vi "DP_WebView_Test.vi"() -> ()   [LabVIEW 2020, in "DP_WebView.lvclass"]
uses:
  DP_WebView.lvclass
  C:/Projects/DependencyViewer/DependencyViewer/DP_WebView_class/data/Microsoft.Web.WebView2.WinForms.dll
  data/Microsoft.Web.WebView2.WinForms.dll
panel:
  in  "Webview container":refnum<k24>(container)
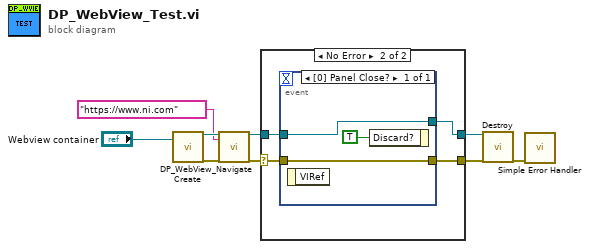
[diagram p0: block diagram]
diagram:
  n1 = call "DP_WebView_Create.vi"("Webview container"="Webview container") -> ("reference out"=w9:refnum<class "DP_WebView.lvclass">, "Error Out"=w8:errorcluster)  [unwired: 11 in, 6 out]
  n2 = call-dynamic "Navigate.vi"("reference in"=w9, "URL"="https://www.ni.com", "Error In"=w8) -> ("reference out"=w7:refnum<class "DP_WebView.lvclass">, "Error Out"=w5:errorcluster)  [unwired: 14 in, 1 out]
  n3 = case shown="No Error" w5 {
    selector: w5 -> [w11 w12]
    tunnel: w7 -> [w10 w15]
    tunnel: [w10 w14] -> w6
    tunnel: [w11 w13] -> w4
    frame Error {
    }
    frame No Error {
      n4 = event shown="[0] Panel Close?" {
        selector: _ -> [_]
        dyn-events: _ -> [_]
        timeout: _ -> [_]
        tunnel: w15 -> [w18]
        tunnel: [w18] -> w14
        tunnel: w12 -> [w17]
        tunnel: [w17] -> w13
        event Panel Close? {
          n5 = event-data() -> ()  [unwired: 1 in, 1 out]
          n6 = event-data("Discard?"=TRUE) -> ()  [unwired: 1 in, 1 out]
        }
      }
    }
  }
  n7 = call-dynamic "Destroy.vi"("reference in"=w6, "Error In"=w4) -> ("Error Out"=w1:errorcluster)  [unwired: 16 in, 1 out]
  n8 = call <vilib>:"Simple Error Handler.vi"("error in (no error)"=w1) -> ()  [unwired: 4 in, 5 out]
